vi "Get Properties of Collection(冲突时的文件备份2013-03-27 14-07-47).vi"(8 "error in (no error)":errorcluster caption="错误输入（无错误）", 11 "ManagementClass 输入":refnum<class "ManagementClass.lvclass"> caption="DNL_LabVIEW Object in") -> (0 "error out":errorcluster caption="错误输出", 1 "非空":bool, 3 "ManagementClass 输出":refnum<class "ManagementClass.lvclass"> caption="DNL_LabVIEW Object out")   [LabVIEW 2012, in "ManagementClass.lvclass"]
uses:
  ManagementClass.lvclass
  ManagementClass.lvclass/ManagementClass.ctl
  System.Management
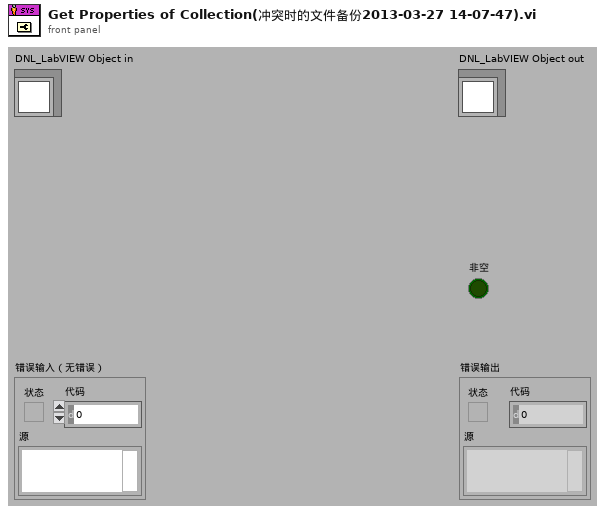
[diagram p1: front panel]
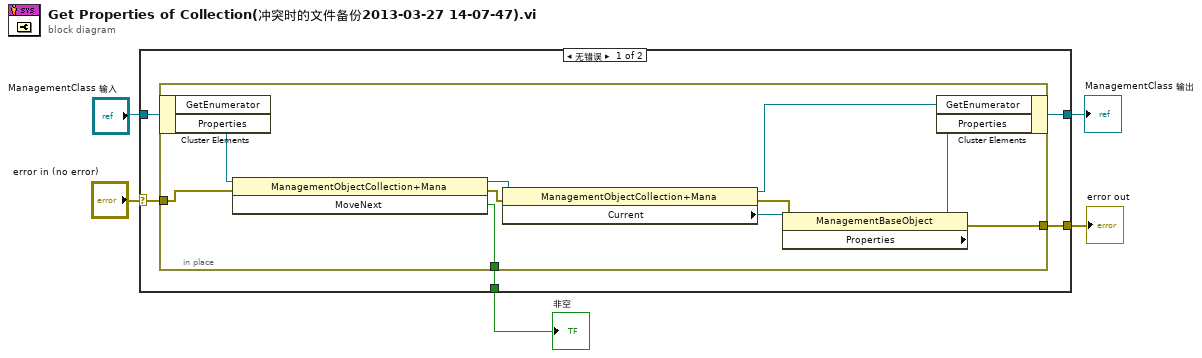
[diagram p0: block diagram]
diagram:
  n1 = case shown="无错误" "error in (no error)" {
    selector: "error in (no error)" -> [w9 w22]
    tunnel: [w7 w22] -> w4
    tunnel: [w8 w21] -> w2
    tunnel: "ManagementClass 输入" -> [w10 w21]
    tunnel: [w6 _] -> w1
    frame No Error {
      n2 = in-place {
        in-place-border: w9 -> [w16]
        in-place-border: [w17] -> w7
        in-place-border: [w14] -> w6
        n3 = in-place-cluster #1(w10) -> ("GetEnumerator"=w15:refnum<k24>)  [unwired: 1 out]
        n4 = invoke class="ManagementObjectCollection+Mana" method="MoveNext"(reference=w15, error in=w16) -> (reference out=w12:refnum<k24>, error out=w13:errorcluster, "MoveNext"=w14:bool)  [unwired: 1 in]
        n5 = property class="ManagementObjectCollection+Mana"(reference=w12, error in=w13) -> (reference out=w11:refnum<k24>, error out=w20:errorcluster, "Current"=w19:refnum<k24>)
        n6 = property class="ManagementBaseObject"(reference=w19, error in=w20) -> (error out=w17:errorcluster, "Properties"=w18:refnum<k24>)  [unwired: 1 out]
        n7 = in-place-cluster #1("GetEnumerator"=w11, "Properties"=w18) -> (w8:refnum<class "ManagementClass.lvclass">)
      }
    }
    frame Error {
    }
  }
  "error out" <- w4
  "ManagementClass 输出" <- w2
  "非空" <- w1
